vi "SR-Test Med System Globals.vi"() -> ()   [LabVIEW 2020]
doc: "This global variable contains all of the strings that are displayed to the user interface or logged to disk by the BoilerMain application."
panel:
  out "Error Logged":string="A critical error occurred.  Check Error Log.txt for more information."
  out "Start Shutdown Purge":string="Start Shutdown Purge"
  out "VI Stopped":string="VI Stopped"
  out "Purge":string="Purge"
  out "Shutdown":string="Shutdown"
  out "Boiler":string="Boiler"
  out "Pilot Decrement (ms)":string="Pilot Decrement (ms)"
  out "Pilot Increment (ms)":string="Pilot Increment (ms)"
  out "Flame Threshold":string="Flame Threshold"
  out "Controller Running":string="Boiler Running"
  out "Forced Draft Fan On":string="Forced Draft Fan On"
  out "Pilot Proved":string="Pilot Proved"
  out "Pilot On":string="Pilot On"
  out "True":string="True"
  out "Purge Time":string="Purge Time"
  out "Controller":string="Controller"
  out "Shutdown Purge Complete":string="Shutdown Purge Complete"
  out "Pre-Purge":string="Pre-Purge"
  out "Start Pre-Purge":string="Start Pre-Purge"
  out "Pre-Purge Complete":string="Pre-Purge Complete"
  out "Ready":string="Ready"
  out "Controller Ready":string="Boiler Ready"
  out "Controller Initialized":string="Boiler Initialized"
  out "Event":string="Event"
  out "Event Data":string="Event Data"
  out "Timestamp":string="Timestamp"
  out "Configuration Files":string="Configuration Files"
  out "MHL":string="MHL"
  out "Fuel Control Valve Minimum":string="Fuel Control Valve Minimum"
  out "Fuel Control Valve Maximum":string="Fuel Control Valve Maximum"
  out "Enter Filename:":string="Select a Boiler INI File:"
  out "Disconnected":string="Lockout"
  # "Status Log Headers"
  # "INI File Strings"
  # "Constants"
  # "Status / Event Strings"
  # "Status Strings"
  # "Event Strings"
  # "Error Logging"
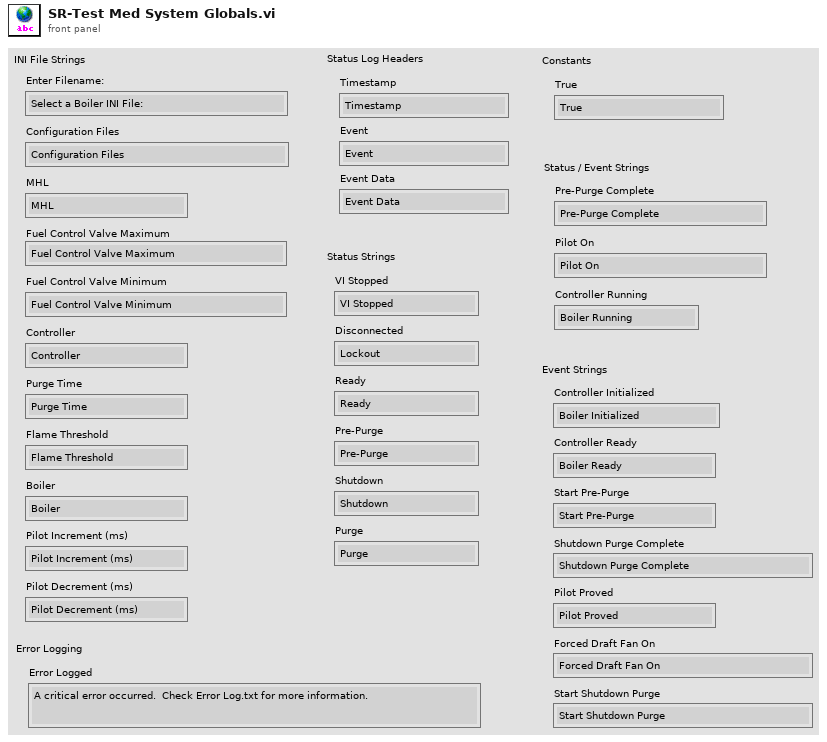
[diagram p1: front panel]
diagram:
